vi "SetParam.vi"(8 "error in (no error)":errorcluster caption="entrée d'erreur (pas d'erreur)", 10 "make_circles":T1={"n_samples"="100", "shuffle"=TRUE, "noise"=-1.0, "random_state"=-1, "factor"=0.8, "Returns"="X"} {"factor" min=0.0 max=1.0; "noise" min=-1.0; "random_state" min=-1}, 11 "Circles.lvclass":refnum<class "Circles.lvclass">) -> (0 "error out":errorcluster caption="sortie d'erreur", 3 "Circles.lvclass":refnum<class "Circles.lvclass">)   [LabVIEW 2020, in "Circles.lvclass"]
doc: "Set Parameters"
uses:
  Circles.lvclass
  Circles.lvclass/Circles.ctl
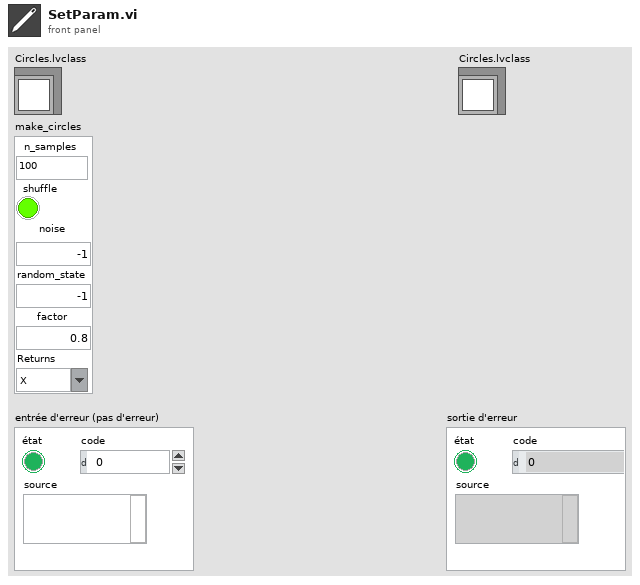
[diagram p1: front panel]
types:
  T1 = cluster{"n_samples":string, "shuffle":bool, "noise":dbl, "random_state":i32, "factor":dbl, "Returns":string}
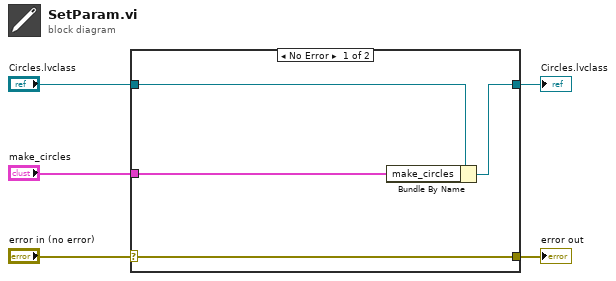
[diagram p0: block diagram]
diagram:
  n1 = case shown="No Error" "error in (no error)" {
    selector: "error in (no error)" -> [w9 w10]
    tunnel: [w9 w10] -> w4
    tunnel: [w7 w11] -> w2
    tunnel: "Circles.lvclass" -> [w8 w11]
    tunnel: "make_circles" -> [w6 _]
    frame No Error {
      n2 = Bundle By Name(cluster=w8, "make_circles"=w6) -> (w7:refnum<class "Circles.lvclass">)
    }
    frame Error {
    }
  }
  "error out" <- w4
  "Circles.lvclass" <- w2
